vi "WLAN DUT Update State Data.vi"(8 "error in (no error)":errorcluster, 11 "niDTS WLAN DUT in":refnum<class "niDTS WLAN Dut.lvclass">) -> (0 "error out":errorcluster, 3 "niDTS WLAN DUT out":refnum<class "niDTS WLAN Dut.lvclass">)   [LabVIEW 2015, in "niDTS WLAN.lvlib" / "niDTS WLAN Dut.lvclass"]
uses:
  niDTS WLAN Dut.lvclass
  niDTS WLAN Dut Data/niDTS WLAN Dut Data.lvclass
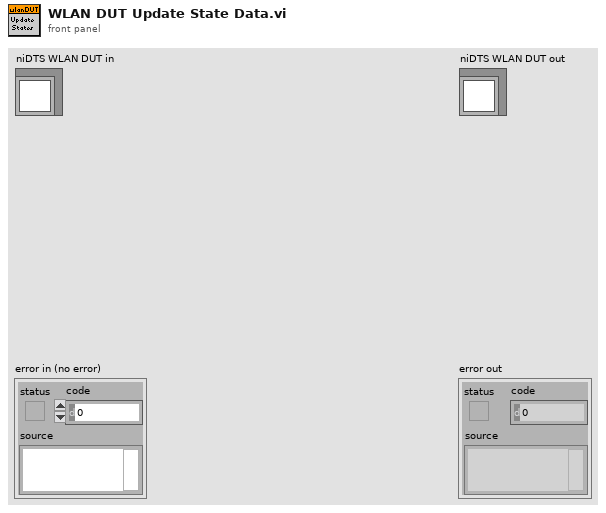
[diagram p1: front panel]
types:
  T1 = typedef "niDTS WLAN.lvlib/niDTS WLAN INC Standard.ctl" = enum16{"802.11 b DSSS", "802.11 a/g OFDM", "802.11 n HT", "802.11 ac VHT"}
  T2 = typedef "niDTS WLAN.lvlib/niDTS WLAN INC CH BW.ctl" = enum16{"20 MHz", "40 MHz", "80 MHz", "160 MHz"}
  T3 = typedef "niDTS WLAN.lvlib/niDTS WLAN INC DSSS Data Rate.ctl" = enum16{"1", "2", "5.5", "11"}
  T4 = typedef "niDTS WLAN.lvlib/niDTS WLAN INC FEC Coding.ctl" = enum16{"BCC", "LDPC"}
  T5 = typedef "niDTS WLAN.lvlib/niDTS WLAN INC GI.ctl" = enum16{"LONG", "SHORT"}
  T6 = typedef "niDTS WLAN.lvlib/niDTS WLAN INC OFDM Data Rate.ctl" = enum16{"6", "9", "12", "18", "24", "36", "48", "54"}
  T7 = typedef "niDTS WLAN.lvlib/niDTS WLAN INC Type.ctl" = enum16{"b - 1 Mbps", "b - 2 Mbps", "b - 5.5 Mbps", "b - 11 Mbps", "ag - 6 Mbps", "ag - 9 Mbps", "ag - 12 Mbps", "ag - 18 Mbps", "ag - 24 Mbps", "ag - 36 Mbps", "ag - 48 Mbps", "ag - 54 Mbps", "n - MCS0", "n - MCS1", "n - MCS2", "n - MCS3", "n - MCS4", "n - MCS5", "n - MCS6", "n - MCS7", "n - MCS8", "n - MCS9", "n - MCS10", "n - MCS11", "n - MCS12", "n - MCS13", "n - MCS14", "n - MCS15", "n - MCS16", "n - MCS17", "n - MCS18", "n - MCS19", "n - MCS20", "n - MCS21", "n - MCS22", "n - MCS23", "n - MCS24", "n - MCS25", "n - MCS26", "n - MCS27", "n - MCS28", "n - MCS29", "n - MCS30", "n - MCS31", "ac - MCS0 -1", "ac - MCS1 -1", "ac - MCS2 -1", "ac - MCS3 -1", "ac - MCS4 -1", "ac - MCS5 -1", "ac - MCS6 -1", "ac - MCS7 -1", "ac - MCS8 -1", "ac - MCS9 -1", "ac - MCS0 -2", "ac - MCS1 -2", "ac - MCS2 -2", "ac - MCS3 -2", "ac - MCS4 -2", "ac - MCS5 -2", "ac - MCS6 -2", "ac - MCS7 -2", "ac - MCS8 -2", "ac - MCS9 -2", "ac - MCS0 -3", "ac - MCS1 -3", "ac - MCS2 -3", "ac - MCS3 -3", "ac - MCS4 -3", "ac - MCS5 -3", "ac - MCS6 -3", "ac - MCS7 -3", "ac - MCS8 -3", "ac - MCS9 -3", "ac - MCS0 -4", "ac - MCS1 -4", "ac - MCS2 -4", "ac - MCS3 -4", "ac - MCS4 -4", "ac - MCS5 -4", "ac - MCS6 -4", "ac - MCS7 -4", "ac - MCS8 -4", "ac - MCS9 -4"}
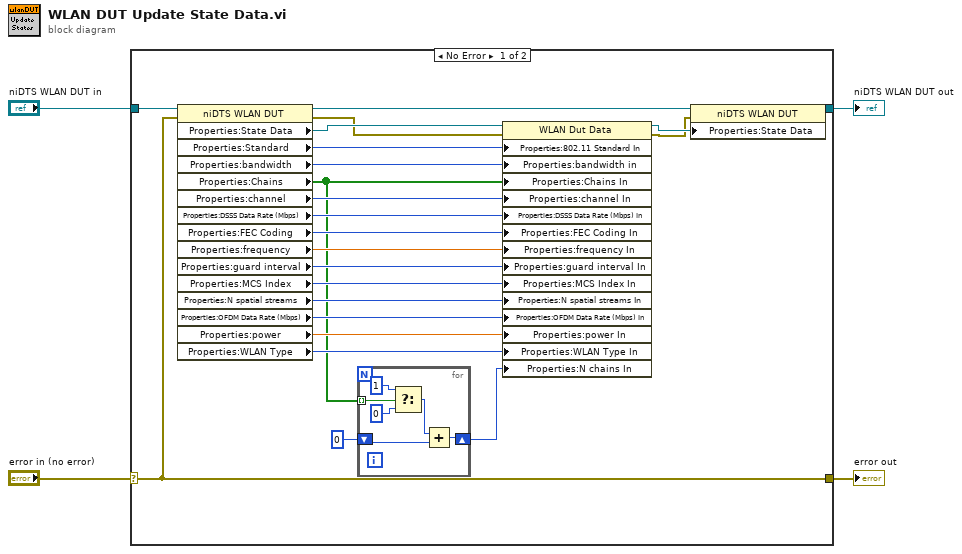
[diagram p0: block diagram]
diagram:
  n1 = case shown="No Error" "error in (no error)" {
    selector: "error in (no error)" -> [w24 w35]
    tunnel: [w24 w35] -> w3
    tunnel: [w25 w34] -> w1
    tunnel: "niDTS WLAN DUT in" -> [w27 w34]
    frame No Error {
      n2 = property class="niDTS WLAN DUT"(reference=w27, error in=w24) -> (reference out=w26:refnum<class "niDTS WLAN Dut.lvclass">, error out=w22:errorcluster, "Properties:State Data"=w23:refnum<class "niDTS WLAN Dut Data.lvclass">, "Properties:Standard"=w21:T1, "Properties:bandwidth"=w20:T2, "Properties:Chains"=w6:bool[], "Properties:channel"=w19:i32, "Properties:DSSS Data Rate (Mbps)"=w18:T3, "Properties:FEC Coding"=w17:T4, "Properties:frequency"=w16:dbl, "Properties:guard interval"=w15:T5, "Properties:MCS Index"=w14:i32, "Properties:N spatial streams"=w13:i32, "Properties:OFDM Data Rate (Mbps)"=w12:T6, "Properties:power"=w11:dbl, "Properties:WLAN Type"=w10:T7)
      n3 = for {
        tunnel: w6 -> [w33] mode=indexing
        shift-right: [w30] -> w5
        shift-left: 0 ("Value") -> [w29]
        n4 = Select(t=1 ("Value"), s=w33, f=0 ("Value")) -> (s? t:f=w28:i32)
        n5 = Add(x=w28, y=w29) -> (x+y=w30:i32)
      }
      n6 = property class="WLAN Dut Data"(reference=w23, error in=w22, "Properties:802.11 Standard In"=w21, "Properties:bandwidth in"=w20, "Properties:Chains In"=w6, "Properties:channel In"=w19, "Properties:DSSS Data Rate (Mbps) In"=w18, "Properties:FEC Coding In"=w17, "Properties:frequency In"=w16, "Properties:guard interval In"=w15, "Properties:MCS Index In"=w14, "Properties:N spatial streams In"=w13, "Properties:OFDM Data Rate (Mbps) In"=w12, "Properties:power In"=w11, "Properties:WLAN Type In"=w10, "Properties:N chains In"=w5) -> (reference out=w9:refnum<class "niDTS WLAN Dut Data.lvclass">, error out=w8:errorcluster)
      n7 = property class="niDTS WLAN DUT"(reference=w26, error in=w8, "Properties:State Data"=w9) -> (reference out=w25:refnum<class "niDTS WLAN Dut.lvclass">)  [unwired: 1 out]
    }
    frame Error {
    }
  }
  "error out" <- w3
  "niDTS WLAN DUT out" <- w1
